vi "Log Error.vi"(8 "error in (no error)":errorcluster, 10 "Error Message Data":T1, 11 "Error Log In":refnum<class "Error Log.lvclass">) -> (0 "error out":errorcluster, 3 "Error Log Out":refnum<class "Error Log.lvclass">)   [LabVIEW 2020, in "Error Log Classes.lvlib" / "Error Log.lvclass"]
uses:
  Error Log.lvclass
  Process Classes/Error Handler/Community/TypeDefs/Error Message Data.ctl
  Process Classes/Error Handler/Error Handler.lvclass
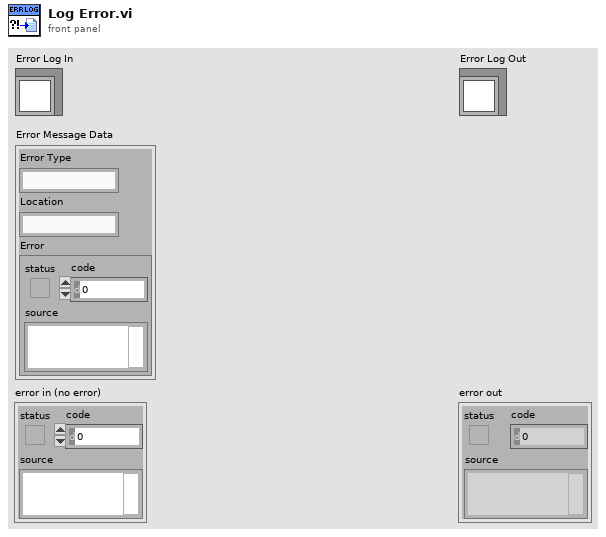
[diagram p1: front panel]
types:
  T1 = typedef "Error Handler.lvclass/Error Message Data.ctl" = cluster{"Error Type":string, "Location":string, "Error":errorcluster}
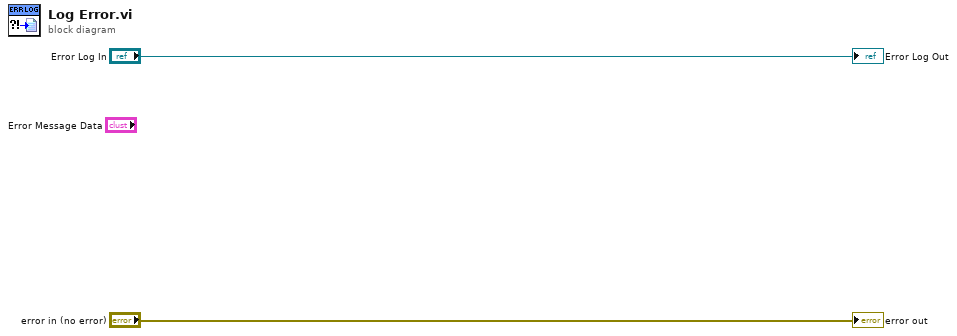
[diagram p0: block diagram]
diagram:
  "error out" <- "error in (no error)"
  "Error Log Out" <- "Error Log In"
